vi "Target Main.vi"() -> ()   [LabVIEW 2021]
uses:
  <vilib>/gmath/NumericalOptimization/stopping criteria.ctl
  <vilib>/Platform/TimedLoop/XDataNode/timing_clust.ctl
  <vilib>/Platform/TimedLoop/XDataNode/nitl_modes.ctl
  <vilib>/Platform/TimedLoop/XDataNode/wakeup.ctl
  <vilib>/Analysis/baseanly.llb/Real Dot Product.vi
  <vilib>/DAQmx/write.llb/DAQmx Write (Digital 1D Bool 1Chan 1Samp).vi
  <vilib>/DAQmx/write.llb/DAQmx Write (Analog 1D DBL NChan 1Samp).vi
  <vilib>/DAQmx/create/channels.llb/DAQmx Create Channel (DO-Digital Output).vi
  <vilib>/DAQmx/create/channels.llb/DAQmx Create Channel (AO-Voltage-Basic).vi
  <vilib>/DAQmx/create/channels.llb/DAQmx Create Channel (AI-Voltage-Basic).vi
  <vilib>/DAQmx/configure/timing.llb/DAQmx Timing (Sample Clock).vi
  <vilib>/DAQmx/miscellaneous.llb/DAQmx Fill In Error Info.vi
  <vilib>/Analysis/Matrix/Numeric/Conversions/Matrix To Array - RM.vi
  <vilib>/platform/TimedLoop/XDataNode/XDataNode.xnode
  <vilib>/Platform/TimedLoop/XDataNode/XDNodeRunTimeDep.lvlib
  <vilib>/Analysis/NI_AALBase.lvlib
  <vilib>/Analysis/Matrix/NI_Matrix.lvlib
  <vilib>/gmath/NI_Gmath.lvlib
panel:
  in  "RBFN On?":bool
  out "RBFN Virtual Spring":dbl
  out "InRange Voltage":dbl[](array[slide]) scale=-5.0..5.0
  out "100ms Finished Late?":bool
  out "100ms":i64=100
  out "1ms Finished Late?":bool
  in  "Tension Control Gains":T1(array[cluster])=[{"proportional gain (Kc)"=0.07, "integral time (Ti, min)"=0.0, "derivative time (Td, min)"=0.0}, {"proportional gain (Kc)"=0.07, "integral time (Ti, min)"=0.0, "derivative time (Td, min)"=0.0}, {"proportional gain (Kc)"=0.07, "integral time (Ti, min)"=0.0, "derivative time (Td, min)"=0.0}] {"derivative time (Td, min)" format="%.3f"; "integral time (Ti, min)" format="%.3f"; "proportional gain (Kc)" format="%.3f"}
  out "1ms":i64=2
  out "10ms Finished Late?":bool
  out "10ms":i64=10
  in  "QP Stopping Criteria":T2={"function tolerance"=0.001, "parameter tolerance"=1e-05, "max iterations"=50, "max function calls"=50, "gradient tolerance"=1e-05, "max time (sec)"=0.01}
  in  "QP?":bool=TRUE
  out "QP Solved":bool=TRUE
  # "TARGET"
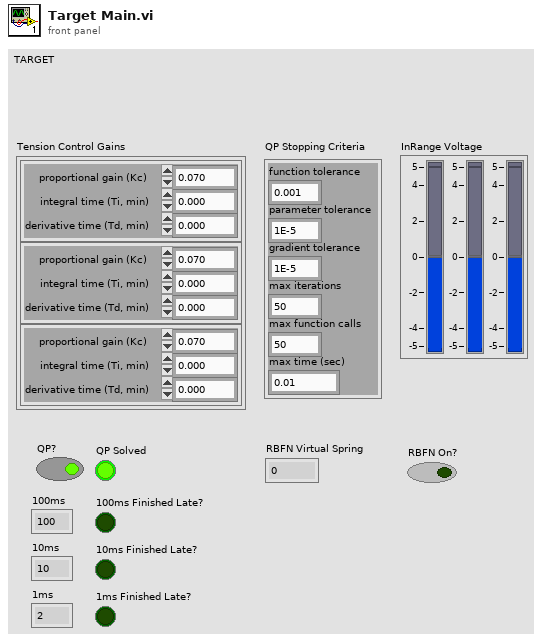
[diagram p1: front panel]
types:
  T1 = cluster{"proportional gain (Kc)":dbl, "integral time (Ti, min)":dbl, "derivative time (Td, min)":dbl}[]
  T2 = typedef "NI_Gmath.lvlib/stopping criteria.ctl" = cluster{"function tolerance":dbl, "parameter tolerance":dbl, "max iterations":i32, "max function calls":i32, "gradient tolerance":dbl, "max time (sec)":dbl}
  T3 = typedef "XDNodeRunTimeDep.lvlib/timing_clust.ctl" = cluster{"Expected End [f-1]":u64, "Actual End [f-1]":u64, "Finished Late? [f-1]":bool, "Expected End [i-1]":u64, "Actual End [i-1]":u64, "Finished Late? [i-1]":bool, "Expected Start [i]":u64, "Actual Start [i]":u64, "Expected Start [f]":u64, "Actual Start [f]":u64, "Source Name":string, "Structure Name":string, "Period":i64, "Deadline":i64, "Offset":i64, "Start":i64, "Priority":i32, "Timeout":i32, "Mode":T4, "Wakeup Reason":T5, "Error":errorcluster, "Source Type":string, "Secondary Source Type":string, "Global End Time":u64, "Global Start Time":u64, "Frame Duration":u64, "Iteration Duration":u64, "Assigned CPU":i32, "I/O Scan Engine Mode":u32}
  T4 = typedef "XDNodeRunTimeDep.lvlib/nitl_modes.ctl" = enum32{"No Change", "Process missed periods, maintain original phase", "Discard missed periods, maintain original phase", "Process missed periods, ignore original phase", "Discard missed periods, ignore original phase"}
  T5 = typedef "XDNodeRunTimeDep.lvlib/wakeup.ctl" = enum32{"Normal", "Aborted", "Asynchronous wakeup", "Timing source error", "Timed loop error", "Timeout"}
  T6 = typedef "NI_Matrix.lvlib/RealMatrix.ctl" = dbl[][]
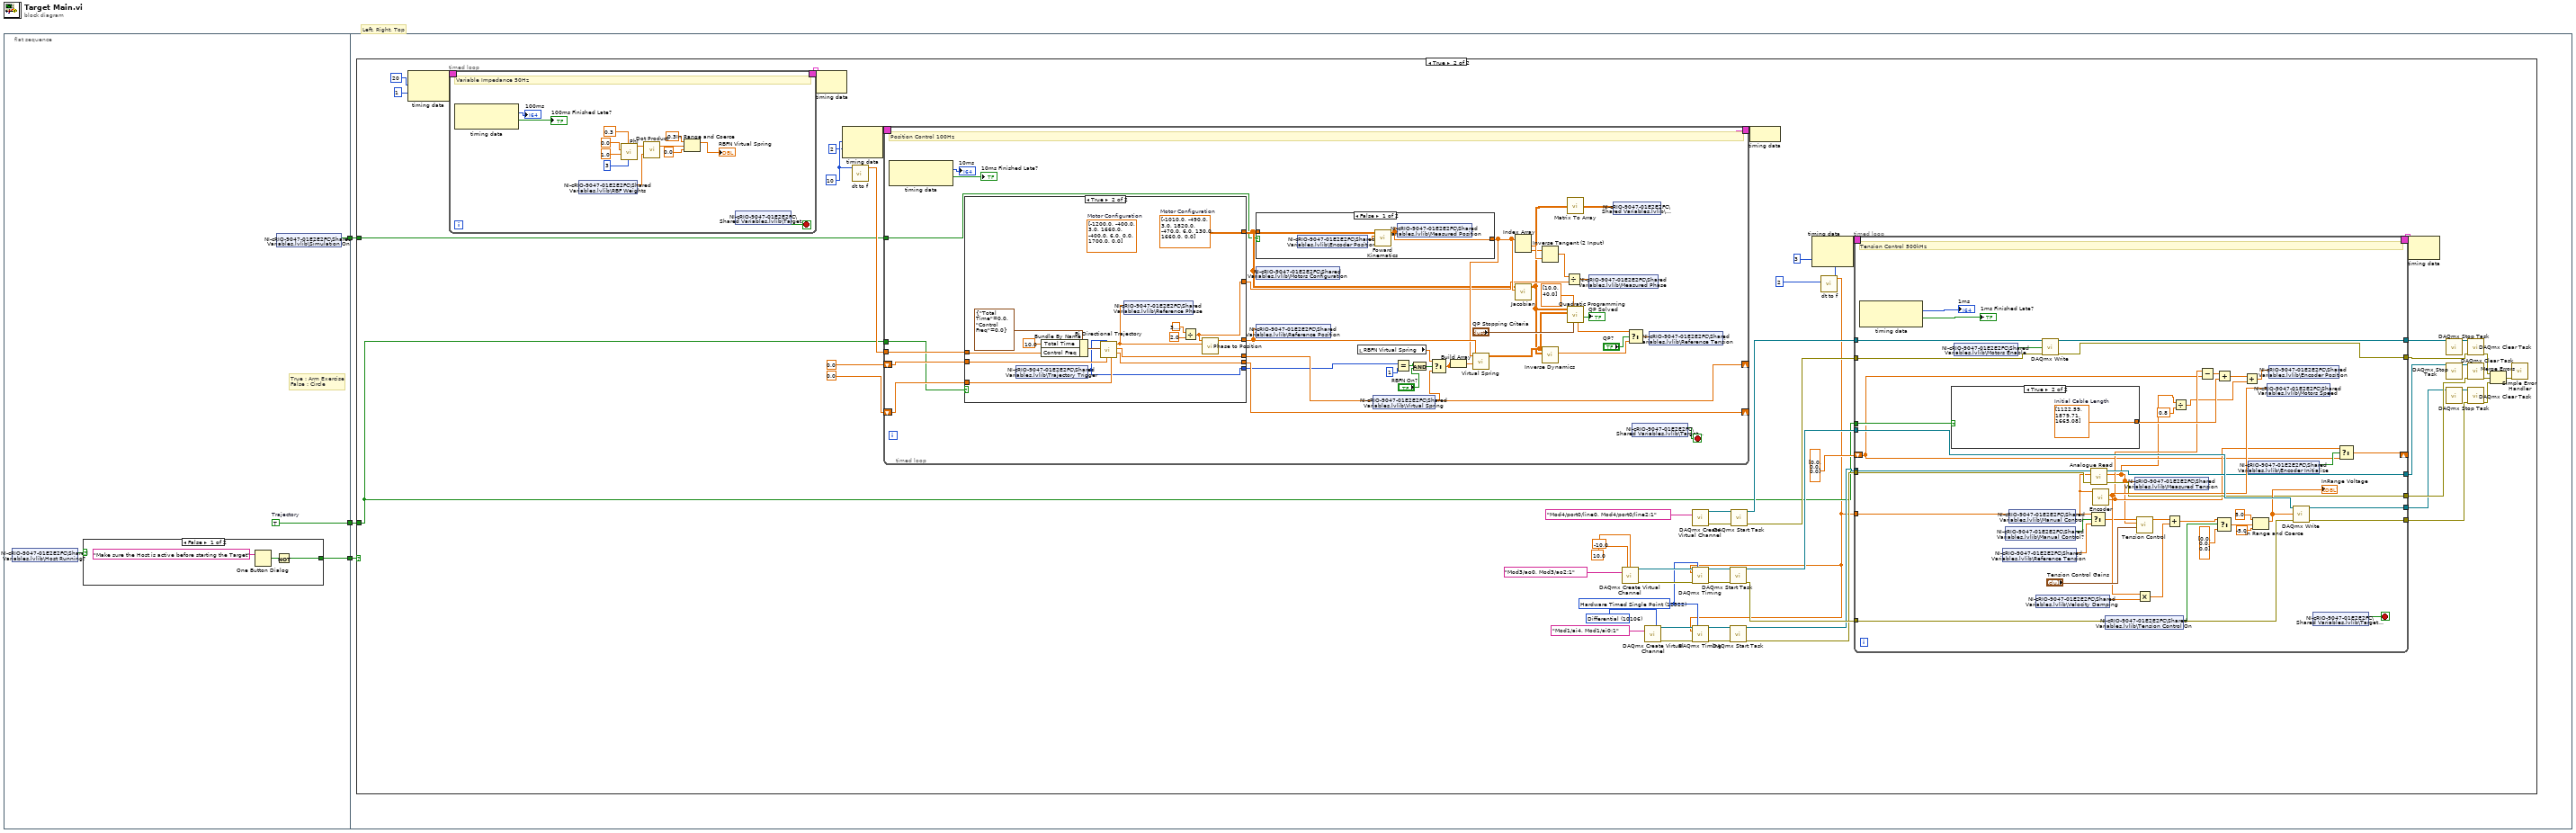
[diagram p0: block diagram]
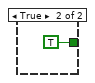
[diagram p2: hidden frame]
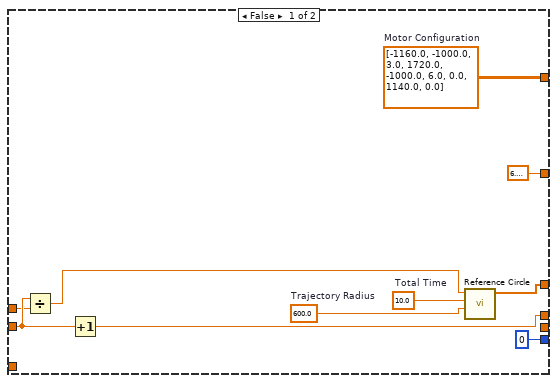
[diagram p4: hidden frame]
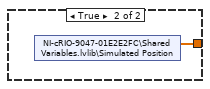
[diagram p5: hidden frame]
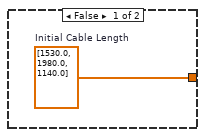
[diagram p6: hidden frame]
diagram:
  # "Left, Right, Top"
  n1 = flat-sequence {
    tunnel: [w6] -> w3
    tunnel: [w5] -> w2
    tunnel: [w4] -> w1
    tunnel: w3 -> [w14]
    tunnel: w2 -> [w13]
    tunnel: w1 -> [w12]
    frame #0 {
      w4 = TRUE  # Trajectory
      # "True : Arm Exercise\nFalse : Circle"
      n2 = shared-variable "NI-cRIO-9047-01E2E2FC\\Shared Variables.lvlib\\Host Running?"() -> (w7:bool)  [unwired: 1 in, 1 out]
      n3 = case shown="False" w7 {
        tunnel: [w8 TRUE] -> w6
        frame False {
          n4 = One Button Dialog(message="Make sure the Host is active before starting the Target") -> (true=w9:bool)  [unwired: 1 in]
          n5 = Not(x=w9) -> (.not. x?=w8:bool)
        }
        frame True {
        }
      }
      n6 = shared-variable "NI-cRIO-9047-01E2E2FC\\Shared Variables.lvlib\\Simulation On"() -> (w5:bool)  [unwired: 1 in, 1 out]
    }
    frame #1 {
      n7 = case shown="True" w14 {
        tunnel: w13 -> [_ w20]
        tunnel: w12 -> [_ w19]
        frame False {
        }
        frame True {
          w27 = i64 10 ("Period 3")
          w26 = 12522 items=["Finite Samples"=10178, "Continuous Samples"=10123, "Hardware Timed Single Point"=12522] ("sample mode")
          w57 = i64 2 ("Period")
          w42 = 10106 items=["Default"=-1, "RSE"=10083, "NRSE"=10078, "Differential"=10106, "Pseudodifferential"=12529] ("input terminal configuration")
          n8 = node-c288(i64 20 ("Period 3"), 1 ("Priority")) -> (w65:T3)
          n9 = timed-loop {
            timing: w65 -> [_]
            timing-out: [_] -> w64
            stop <- w72 stop-if-true
            # "Variable Impedance 50Hz"
            n10 = node-c288() -> (→"100ms":i64, →"100ms Finished Late?":bool)  [unwired: 1 in]
            n11 = shared-variable "NI-cRIO-9047-01E2E2FC\\Shared Variables.lvlib\\RBF Weights"() -> (w71:dbl[])  [unwired: 1 in, 1 out]
            n12 = call "Phi.vi"("Number"=3, "STD"=0.3, "x_f"=1.0, "x_0"=0.0) -> ("Array"=w80:dbl[])  [unwired: 7 in]
            n13 = call-poly <vilib>:"Dot Product.vi"("Y Vector"=w71, "X Vector"=w80) -> ("X * Y"=w79:dbl)  [unwired: 1 out]
            n14 = In Range and Coerce(upper limit=0.3, x=w79, lower limit=0.0) -> (coerced(x)=→"RBFN Virtual Spring":dbl)  [unwired: 1 out]
            n15 = shared-variable "NI-cRIO-9047-01E2E2FC\\Shared Variables.lvlib\\Target Stop"() -> (w72:bool)  [unwired: 1 in, 1 out]
          }
          n16 = node-c288(w64) -> ()  [unwired: 1 out]
          n17 = node-c288(w27, 2 ("Priority")) -> (w67:T3)
          n18 = call "dt to f.vi"("Period"=w27) -> ("Frequency"=w23:dbl)  [unwired: 10 in]
          n19 = timed-loop {
            timing: w67 -> [_]
            timing-out: [_] -> w66
            tunnel: w23 -> [w113]
            shift-right: [w116] -> _
            shift-left: 0.0 ("Go Next Time") -> [w118]
            shift-right: [w115] -> _
            shift-left: 0.0 ("Return Next Time") -> [w117]
            tunnel: w20 -> [w105]
            tunnel: w19 -> [w104]
            stop <- w103 stop-if-true
            # "Position Control 100Hz"
            n20 = node-c288() -> (→"10ms":i64, →"10ms Finished Late?":bool)  [unwired: 1 in]
            n21 = case shown="True" w104 {
              tunnel: w118 -> [w140 w151]
              tunnel: w117 -> [_ w150]
              tunnel: [w141 w149] -> w116
              tunnel: [_ w148] -> w115
              tunnel: [w134 w147] -> w114
              tunnel: w113 -> [w139 w146]
              tunnel: [6.283185307179586 w144] -> w107
              tunnel: [w135 w143] -> w106
              tunnel: [0 w142] -> w102
              frame False {
                w137 = 600.0  # Trajectory Radius
                w135 = dbl[][] [[-1160.0, -1000.0, 3.0], [1720.0, -1000.0, 6.0], [0.0, 1140.0, 0.0]]  # Motor Configuration
                w138 = 10.0  # Total Time
                n22 = Divide(x=w140, y=w139) -> (x/y=w136:dbl)
                n23 = Increment(x=w140) -> (x+1=w141:dbl)
                n24 = call "Reference Circle.vi"("Radius"=w137, "Frequency"=w138, "Time"=w136) -> ("Reference Position"=w134:dbl[])  [unwired: 8 in]
              }
              frame True {
                (unwired) dbl[][] [[-1200.0, -400.0, 3.0], [1660.0, -400.0, 6.0], [0.0, 1700.0, 0.0]]  # Motor Configuration
                w143 = dbl[][] [[-1010.0, -490.0, 3.0], [1820.0, -470.0, 6.0], [130.0, 1660.0, 0.0]]  # Motor Configuration
                n25 = shared-variable "NI-cRIO-9047-01E2E2FC\\Shared Variables.lvlib\\Trajectory Trigger"() -> (w142:i32)  [unwired: 1 in, 1 out]
                n26 = Bundle By Name(cluster=cluster{"Total Time":dbl, "Control Freq":dbl} {"Total Time"=0.0, "Control Freq"=0.0} ("input cluster"), "Total Time"=10.0, "Control Freq"=w146) -> (w152:cluster{"Total Time":dbl, "Control Freq":dbl})
                n27 = call "Bi Directional Trajectory.vi"("Return Time"=w150, "Go Time"=w151, "Traj Start"=w142, "Trajectory Settings"=w152) -> ("Return Next Time"=w148:dbl, "Go Next Time"=w149:dbl, "Phase"=w145:dbl)  [unwired: 5 in]
                n28 = shared-variable "NI-cRIO-9047-01E2E2FC\\Shared Variables.lvlib\\Reference Phase"(w145) -> ()  [unwired: 1 in, 1 out]
                n29 = Divide(x=3.141592653589793, y=2.0) -> (x/y=w144:dbl)
                n30 = call "Phase to Position.vi"("Phase"=w145, "Total Angle"=w144) -> ("x,y"=w147:dbl[])  [unwired: 9 in]
              }
            }
            n31 = case shown="False" w105 {
              tunnel: [w158 w160] -> w108
              tunnel: w106 -> [w157 _]
              frame False {
                n32 = shared-variable "NI-cRIO-9047-01E2E2FC\\Shared Variables.lvlib\\Encoder Position"() -> (w159:dbl[])  [unwired: 1 in, 1 out]
                n33 = call "Foward Kinematics.vi"("Encoder Position"=w159, "Motor Configuration"=w157) -> ("Measured Position"=w158:dbl[])  [unwired: 9 in]
                n34 = shared-variable "NI-cRIO-9047-01E2E2FC\\Shared Variables.lvlib\\Measured Position"(w158) -> ()  [unwired: 1 in, 1 out]
              }
              frame True {
                n35 = shared-variable "NI-cRIO-9047-01E2E2FC\\Shared Variables.lvlib\\Simulated Position"() -> (w160:dbl[])  [unwired: 1 in, 1 out]
              }
            }
            n36 = shared-variable "NI-cRIO-9047-01E2E2FC\\Shared Variables.lvlib\\Motors Configuration"(w106) -> ()  [unwired: 1 in, 1 out]
            n37 = shared-variable "NI-cRIO-9047-01E2E2FC\\Shared Variables.lvlib\\Reference Position"(w114) -> ()  [unwired: 1 in, 1 out]
            n38 = local read "RBFN Virtual Spring"() -> (w100:dbl)
            n39 = shared-variable "NI-cRIO-9047-01E2E2FC\\Shared Variables.lvlib\\Virtual Spring"() -> (w95:dbl)  [unwired: 1 in, 1 out]
            n40 = Equal?(x=w102, y=1) -> (x = y?=w94:bool)
            n41 = And(x=w94, y="RBFN On?") -> (x .and. y?=w93:bool)
            n42 = Select(t=w100, s=w93, f=w95) -> (s? t:f=w99:dbl)
            n43 = Build Array(w99, w99) -> (w98:dbl[])
            n44 = call "Virtual Spring.vi"("P Gain"=w98, "Reference Position"=w114, "Actual Position"=w108) -> ("Desired Force Matrix"=w125:T6)  [unwired: 8 in]
            n45 = Index Array(array=w108) -> (element #1=w112:dbl, element #2=w111:dbl)  [unwired: 2 in]
            n46 = call "Jacobian.vi"("EE Position"=w108, "Motor Configuration"=w106) -> ("Jacobian"=w97:T6)  [unwired: 9 in]
            n47 = Inverse Tangent (2 Input)(1:w112, 2:w111) -> (0:w110:dbl)
            n48 = call "Inverse Dynamics.vi"("Jacobian Matrix"=w97, "F desired Matrix"=w125) -> ("Reference Tension"=w124:dbl[])  [unwired: 9 in]
            n49 = Divide(x=w110, y=w107) -> (x/y=w109:dbl)
            n50 = call-poly <vilib>:"Matrix To Array.vi"("Real Matrix"=w97) -> ("Real 2D Array"=w96:dbl[][])
            n51 = call "Quadratic Programming.vi"("stopping Criteria"="QP Stopping Criteria", "UB"=dbl[] [10.0, 40.0] ("LB"), "Desired Force Matrix"=w125, "Jacobian"=w97) -> ("Boolean"=→"QP Solved":bool, "minimum"=w123:dbl[])  [unwired: 4 in, 2 out]
            n52 = shared-variable "NI-cRIO-9047-01E2E2FC\\Shared Variables.lvlib\\Measured Phase"(w109) -> ()  [unwired: 1 in, 1 out]
            n53 = shared-variable "NI-cRIO-9047-01E2E2FC\\Shared Variables.lvlib\\Jacobian"(w96) -> ()  [unwired: 1 in, 1 out]
            n54 = Select(t=w123, s="QP?", f=w124) -> (s? t:f=w121:dbl[])
            n55 = shared-variable "NI-cRIO-9047-01E2E2FC\\Shared Variables.lvlib\\Target Stop"() -> (w103:bool)  [unwired: 1 in, 1 out]
            n56 = shared-variable "NI-cRIO-9047-01E2E2FC\\Shared Variables.lvlib\\Reference Tension"(w121) -> ()  [unwired: 1 in, 1 out]
          }
          n57 = call-poly <vilib>:"DAQmx Create Virtual Channel.vi"("maximum value"=10.0 ("AO max"), "minimum value"=-10.0 ("AO min"), "physical channels"=tag "Mod3/ao0, Mod3/ao2:1" ("Physical Channel(s)")) -> ("task out"=w49:refnum<k21>, "error out"=w51:errorcluster)  [unwired: 11 in]
          n58 = call-poly <vilib>:"DAQmx Create Virtual Channel.vi"("input terminal configuration"=w42, "physical channels"=tag "Mod1/ai4, Mod1/ai0:1") -> ("task out"=w53:refnum<k21>, "error out"=w55:errorcluster)  [unwired: 12 in]
          n59 = call-poly <vilib>:"DAQmx Create Virtual Channel.vi"("lines"=tag "Mod4/port0/line0, Mod4/port0/line2:1") -> ("task out"=w48:refnum<k21>, "error out"=w47:errorcluster)  [unwired: 13 in]
          n60 = call <vilib>:"DAQmx Start Task.vi"("task/channels in"=w48, "error in"=w47) -> ("task out"=w61:refnum<k21>, "error out"=w60:errorcluster)  [unwired: 12 in]
          n61 = node-c288(w66) -> ()
          n62 = node-c288(w57, 3 ("Priority")) -> (w69:T3)
          n63 = call "dt to f.vi"("Period"=w57) -> ("Frequency"=w15:dbl)  [unwired: 10 in]
          n64 = call-poly <vilib>:"DAQmx Timing.vi"("task/channels in"=w49, "sample mode"=w26, "rate"=w15, "error in"=w51) -> ("task out"=w50:refnum<k21>, "error out"=w52:errorcluster)  [unwired: 10 in]
          n65 = call-poly <vilib>:"DAQmx Timing.vi"("task/channels in"=w53, "sample mode"=w26, "rate"=w15, "error in"=w55) -> ("task out"=w54:refnum<k21>, "error out"=w56:errorcluster)  [unwired: 10 in]
          n66 = call <vilib>:"DAQmx Start Task.vi"("task/channels in"=w50, "error in"=w52) -> ("task out"=w63:refnum<k21>, "error out"=w62:errorcluster)  [unwired: 12 in]
          n67 = call <vilib>:"DAQmx Start Task.vi"("task/channels in"=w54, "error in"=w56) -> ("task out"=w59:refnum<k21>, "error out"=w58:errorcluster)  [unwired: 12 in]
          n68 = timed-loop {
            tunnel: [w182] -> w31
            tunnel: [w181] -> w34
            tunnel: [w184] -> w33
            tunnel: [w183] -> w35
            tunnel: w59 -> [w209]
            tunnel: w58 -> [w208]
            tunnel: w63 -> [w205]
            tunnel: w62 -> [w210]
            tunnel: w61 -> [w207]
            tunnel: w60 -> [w206]
            tunnel: [w186] -> w29
            shift-right: [w174] -> _
            shift-left: dbl[] [0.0, 0.0, 0.0] ("Encoder Position (mm)") -> [w172]
            timing: w69 -> [_]
            timing-out: [_] -> w68
            tunnel: w15 -> [w179]
            tunnel: [w185] -> w36
            tunnel: w19 -> [w175]
            stop <- w171 stop-if-true
            # "Tension Control 500kHz"
            n69 = node-c288() -> (→"1ms":i64, →"1ms Finished Late?":bool)  [unwired: 1 in]
            n70 = case shown="True" w175 {
              tunnel: [w211 w212] -> w177
              frame False {
                w211 = dbl[] [1530.0, 1980.0, 1140.0]  # Initial Cable Length
              }
              frame True {
                w212 = dbl[] [1122.59, 1879.71, 1665.08]  # Initial Cable Length
              }
            }
            n71 = shared-variable "NI-cRIO-9047-01E2E2FC\\Shared Variables.lvlib\\Motors Enable"() -> (w200:bool[])  [unwired: 1 in, 1 out]
            n72 = shared-variable "NI-cRIO-9047-01E2E2FC\\Shared Variables.lvlib\\Reference Tension"() -> (w176:dbl[])  [unwired: 1 in, 1 out]
            n73 = shared-variable "NI-cRIO-9047-01E2E2FC\\Shared Variables.lvlib\\Manual Control?"() -> (w188:bool)  [unwired: 1 in, 1 out]
            n74 = shared-variable "NI-cRIO-9047-01E2E2FC\\Shared Variables.lvlib\\Manual Control"() -> (w187:dbl[])  [unwired: 1 in, 1 out]
            n75 = shared-variable "NI-cRIO-9047-01E2E2FC\\Shared Variables.lvlib\\Velocity Damping"() -> (w196:dbl)  [unwired: 1 in, 1 out]
            n76 = call-poly <vilib>:"DAQmx Write.vi"("task/channels in"=w207, "data"=w200, "error in"=w206) -> ("task out"=w186:refnum<k21>, "error out"=w185:errorcluster)  [unwired: 10 in, 1 out]
            n77 = Select(t=w187, s=w188, f=w176) -> (s? t:f=w189:dbl[])
            n78 = call "Analogue Read.vi"("error in"=w208, "sampling freq: fs"=w179, "task/channels in"=w209) -> ("error out"=w183:errorcluster, "Measured Tension"=w168:dbl[], "task out"=w184:refnum<k21>)  [unwired: 6 in]
            n79 = call "Encoder.vi"("Frequency"=w179) -> ("Encoder Position (mm)"=w173:dbl[], "RPM"=w190:dbl[])  [unwired: 9 in]
            n80 = shared-variable "NI-cRIO-9047-01E2E2FC\\Shared Variables.lvlib\\Tension Control On"() -> (w191:bool)  [unwired: 1 in, 1 out]
            n81 = shared-variable "NI-cRIO-9047-01E2E2FC\\Shared Variables.lvlib\\Measured Tension"(w168) -> ()  [unwired: 1 in, 1 out]
            n82 = call "Tension Control.vi"("PID gains"="Tension Control Gains", "Measured Tension"=w168, "Reference Tension"=w189) -> ("Voltage Output"=w195:dbl[])  [unwired: 8 in]
            n83 = Multiply(x=w190, y=w196) -> (x*y=w193:dbl[])
            n84 = Add(x=w195, y=w193) -> (x+y=w194:dbl[])
            n85 = Divide(x=w168, y=0.8) -> (x/y=w167:dbl[])
            n86 = Subtract(x=w173, y=w172) -> (x-y=w178:dbl[])
            n87 = Select(t=w194, s=w191, f=dbl[] [0.0, 0.0, 0.0]) -> (s? t:f=w202:dbl[])
            n88 = Add(x=w178, y=w177) -> (x+y=w170:dbl[])
            n89 = Add(x=w170, y=w167) -> (x+y=w169:dbl[])
            n90 = shared-variable "NI-cRIO-9047-01E2E2FC\\Shared Variables.lvlib\\Encoder Initialize"() -> (w201:bool)  [unwired: 1 in, 1 out]
            n91 = In Range and Coerce(upper limit=5.0, x=w202, lower limit=-5.0) -> (coerced(x)=w199:dbl[])  [unwired: 1 out]
            "InRange Voltage" <- w199
            n92 = shared-variable "NI-cRIO-9047-01E2E2FC\\Shared Variables.lvlib\\Motors Speed"(w190) -> ()  [unwired: 1 in, 1 out]
            n93 = shared-variable "NI-cRIO-9047-01E2E2FC\\Shared Variables.lvlib\\Encoder Position"(w169) -> ()  [unwired: 1 in, 1 out]
            n94 = call-poly <vilib>:"DAQmx Write.vi"("task/channels in"=w205, "data"=w199, "error in"=w210) -> ("task out"=w182:refnum<k21>, "error out"=w181:errorcluster)  [unwired: 10 in, 1 out]
            n95 = shared-variable "NI-cRIO-9047-01E2E2FC\\Shared Variables.lvlib\\Target Stop"() -> (w171:bool)  [unwired: 1 in, 1 out]
            n96 = Select(t=w173, s=w201, f=w172) -> (s? t:f=w174:dbl[])
          }
          n97 = node-c288(w68) -> ()  [unwired: 1 out]
          n98 = call <vilib>:"DAQmx Stop Task.vi"("task/channels in"=w29) -> ("task out"=w28:refnum<k21>)  [unwired: 13 in, 1 out]
          n99 = call <vilib>:"DAQmx Stop Task.vi"("task/channels in"=w33) -> ("task out"=w32:refnum<k21>)  [unwired: 13 in, 1 out]
          n100 = call <vilib>:"DAQmx Stop Task.vi"("task/channels in"=w31) -> ("task out"=w30:refnum<k21>)  [unwired: 13 in, 1 out]
          n101 = call <vilib>:"DAQmx Clear Task.vi"("task in"=w28, "error in"=w36) -> ("error out"=w40:errorcluster)  [unwired: 13 in]
          n102 = call <vilib>:"DAQmx Clear Task.vi"("task in"=w32, "error in"=w35) -> ("error out"=w39:errorcluster)  [unwired: 13 in]
          n103 = call <vilib>:"DAQmx Clear Task.vi"("task in"=w30, "error in"=w34) -> ("error out"=w38:errorcluster)  [unwired: 13 in]
          n104 = Merge Errors(w40, w39, w38) -> (w37:errorcluster)
          n105 = call <vilib>:"Simple Error Handler.vi"("error in (no error)"=w37) -> ()  [unwired: 4 in, 5 out]
        }
      }
    }
  }
